vi "InitCommentLog.vi"(8 "error control":errorcluster, 11 "file path (use dialog)":path) -> (0 "error indicator":errorcluster, 3 "refnum out":refnum<file>)   [LabVIEW 2014]
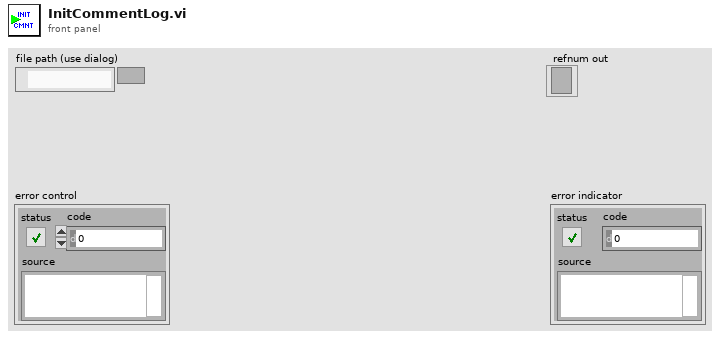
[diagram p1: front panel]
types:
  T1 = enum16{"open", "replace", "create", "open or create", "replace or create", "replace or create with confirmation"}
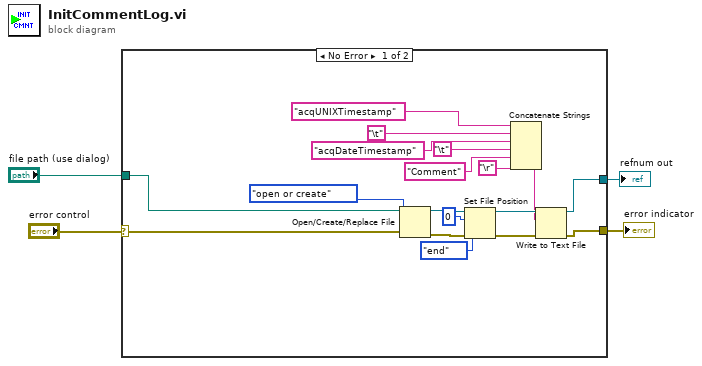
[diagram p0: block diagram]
diagram:
  n1 = case shown="No Error" "error control" {
    selector: "error control" -> [w6 w23]
    tunnel: [w8 w23] -> w3
    tunnel: [w7 _] -> w2
    tunnel: "file path (use dialog)" -> [w5 _]
    frame No Error {
      n2 = Open/Create/Replace File(file path (use dialog)=w5, error in=w6, operation (0:open)=T1."open or create") -> (refnum out=w20:refnum<file>, error out=w17:errorcluster)  [unwired: 3 in, 1 out]
      n3 = Set File Position(offset (in bytes) (0)=i64 0, refnum=w20, from (0:start)=enum16{"start", "end", "current"}."end", error in=w17) -> (refnum out=w19:refnum<file>, error out=w18:errorcluster)
      n4 = Concatenate Strings("acqUNIXTimestamp" ("string"), "\t", "acqDateTimestamp" ("string"), "\t", "Comment" ("string"), "\r") -> (w15:string)
      n5 = Write to Text File(file (use dialog)=w19, text=w15, error in=w18) -> (refnum out=w7:refnum<file>, error out=w8:errorcluster)  [unwired: 1 in, 1 out]
    }
    frame Error {
    }
  }
  "error indicator" <- w3
  "refnum out" <- w2
